vi "tempcorrectchannelname.vi"(1 "param in":T1, 2 "command":string) -> (0 "param out":T1)   [LabVIEW 2015]
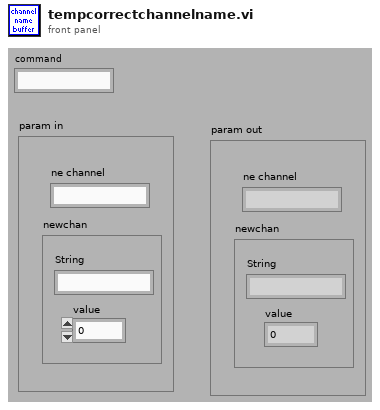
[diagram p1: front panel]
types:
  T1 = cluster{"newchan":cluster{"String":string, "value":i32}, "ne channel":string}
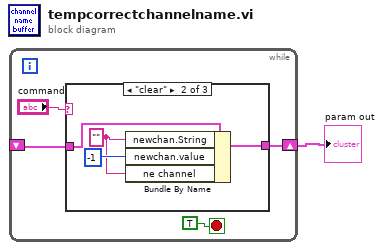
[diagram p0: block diagram]
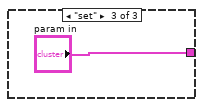
[diagram p3: hidden frame]
diagram:
  n1 = while {
    shift-right: [w3] -> w1
    shift-left: _ -> [w2]
    stop <- TRUE stop-if-true
    n2 = case shown="\"clear\"" "command" {
      tunnel: [w6 w10 "param in"] -> w3
      tunnel: w2 -> [w6 w9 _]
      frame "get", Default {
      }
      frame "clear" {
        w7 = "" ("String")
        n3 = Bundle By Name(cluster=w9, "newchan.String"=w7, "newchan.value"=-1 ("value"), "ne channel"=w7) -> (w10:T1)
      }
      frame "set" {
      }
    }
  }
  "param out" <- w1
